vi "Turret_Globals.vi"() -> ()   [LabVIEW 2019]
uses:
  Turret_Cluster.ctl
  Turret_States.ctl
panel:
  in  "Turret_Execute_Notifier":refnum<notifier>
  in  "Turret_Set_Notifier":refnum<notifier>
  out "Turret_Locked":bool
  out "Turret_Is_Corrected":bool
  in  "Turret_Wraparound":dbl
  in  "Turret_CANcoder":string="Turret_CANcoder"
  in  "Turret_Spin":string="Turret_Spin"
  in  "Turret_Execute_Ref":string="Turret_Execute_Ref"
  in  "Turret_Set_Ref":string="Turret_Set_ref"
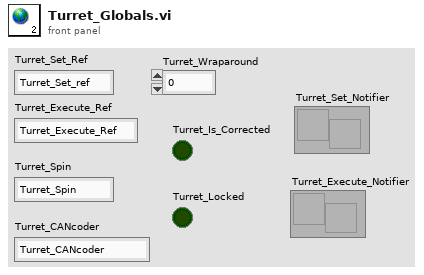
[diagram p1: front panel]
diagram:
